vi "Launcher - TCP Client Example.vi"(6 "Worker Alias":string="TCP Client Example", 8 "error in":errorcluster, 9 "Initialization Data":T1, 11 "TCP Client Example in":refnum<class "TCP Client Example.lvclass">) -> (0 "error out":errorcluster)   [LabVIEW 2017]
doc: "This VI launches the Head Worker of a Workers application."
uses:
  Workers/TCP Client Example/Initialization Data.ctl
  Workers/TCP Client Example/TCP Client Example.lvclass
  C:/SC/Source Code/VIPM/LabVIEW 20xx/vi.lib/addons/_Workers/Library/Classes/Worker/Worker.lvclass
  <vilib>/addons/_Workers/Debugger/Debug Client/Debug Client.lvlib
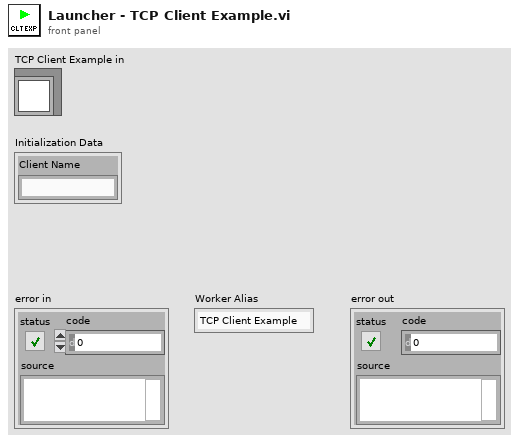
[diagram p1: front panel]
types:
  T1 = typedef "TCP Client Example.lvclass/Initialization Data.ctl" = cluster{"Client Name":string}
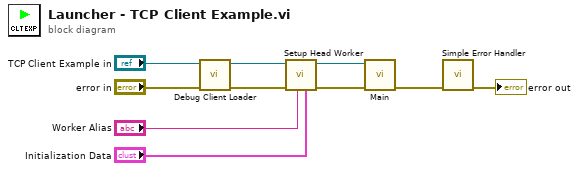
[diagram p0: block diagram]
diagram:
  n1 = call <vilib>:"Debug Client Loader.vi"("error in (no error)"="error in", "Worker_"="TCP Client Example in") -> ("error out"=w3:errorcluster, "Worker_out"=w1:refnum<class "TCP Client Example.lvclass">)  [unwired: 8 in]
  n2 = call-dynamic "Setup Head Worker.vi"("Initalization Data"="Initialization Data", "Worker Alias"="Worker Alias", "error in"=w3, "Worker_"=w1) -> ("error out"=w10:errorcluster, "Worker_out"=w7:refnum<class "TCP Client Example.lvclass">)  [unwired: 6 in]
  n3 = call-dynamic "Main.vi"("error in"=w10, "TCP Client Example in"=w7) -> ("error out"=w8:errorcluster)  [unwired: 8 in, 1 out]
  n4 = call <vilib>:"Simple Error Handler.vi"("error in (no error)"=w8) -> ("error out"=→"error out":errorcluster)  [unwired: 4 in, 4 out]
